vi "Get Handlers.vi"(8 "error in":errorcluster, 11 "Logger in":refnum<class "Logger.lvclass">) -> (0 "error out":errorcluster, 2 "Handlers":refnum<class "Handler.lvclass">[](array[class]), 3 "Logger out":refnum<class "Logger.lvclass">)   [LabVIEW 2016, in "hse-logger.lvlib" / "Logger.lvclass"]
doc: "Returns an array of all Handlers in this logger."
uses:
  Logger.lvclass
  Handler/Handler.lvclass
  Logger.lvclass/Logger.ctl
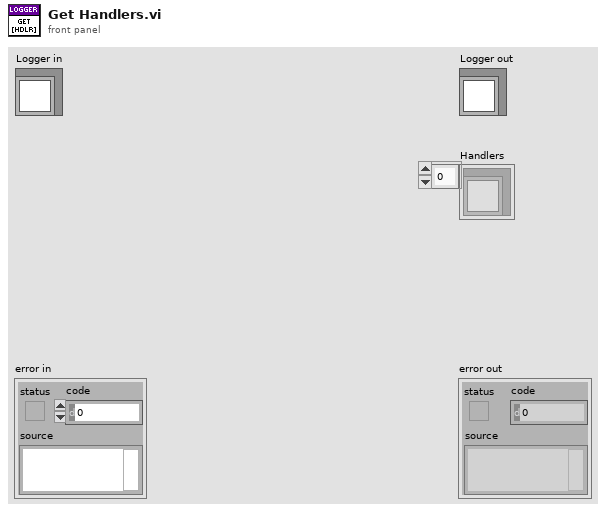
[diagram p1: front panel]
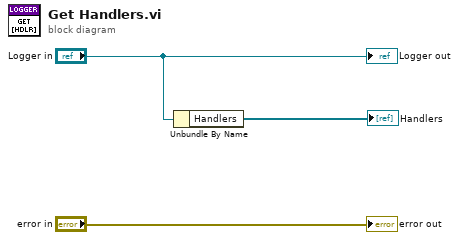
[diagram p0: block diagram]
diagram:
  n1 = Unbundle By Name("Logger in") -> ("Handlers"=→"Handlers":refnum<class "Handler.lvclass">[])
  "error out" <- "error in"
  "Logger out" <- "Logger in"
